vi "pruebas con Alarm Log y Fill Table.vi"() -> ()   [LabVIEW 2018]
panel:
  in  "Filtrar por Alarma?":bool
  out "Array":string[][](array[string])
  out "Real Time Alarms (last 100 records)":i32(listbox)
  out "RT Alarm Log":string[](array[string])
  out "Numeric":i32
  out "PQ_Log array out":i16[](array[numeric])
  out "Boolean array 6":bool[](array[boolean])
  in  "stop":bool
  # "Sag_Indication_Detected"
  # "Swell_Indication_Detected"
  # "Transient_Indication"
  # "200mS_Sag_Swell_Status_Flag"
  # "3s_Sag_Swell_Status_Flag"
  # "10m_Sag_Swell_Status_Flag"
  # "2h_Sag_Swell_Status_Flag"
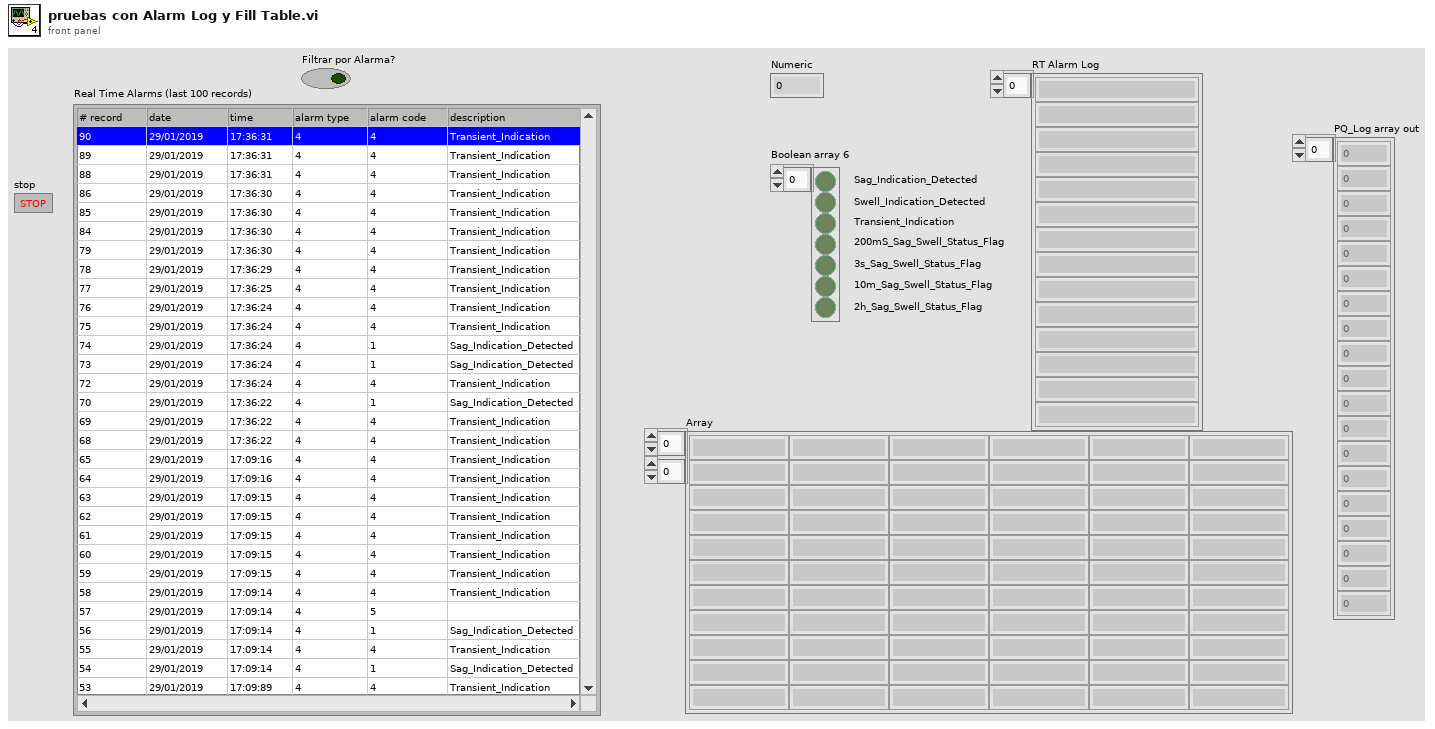
[diagram p1: front panel]
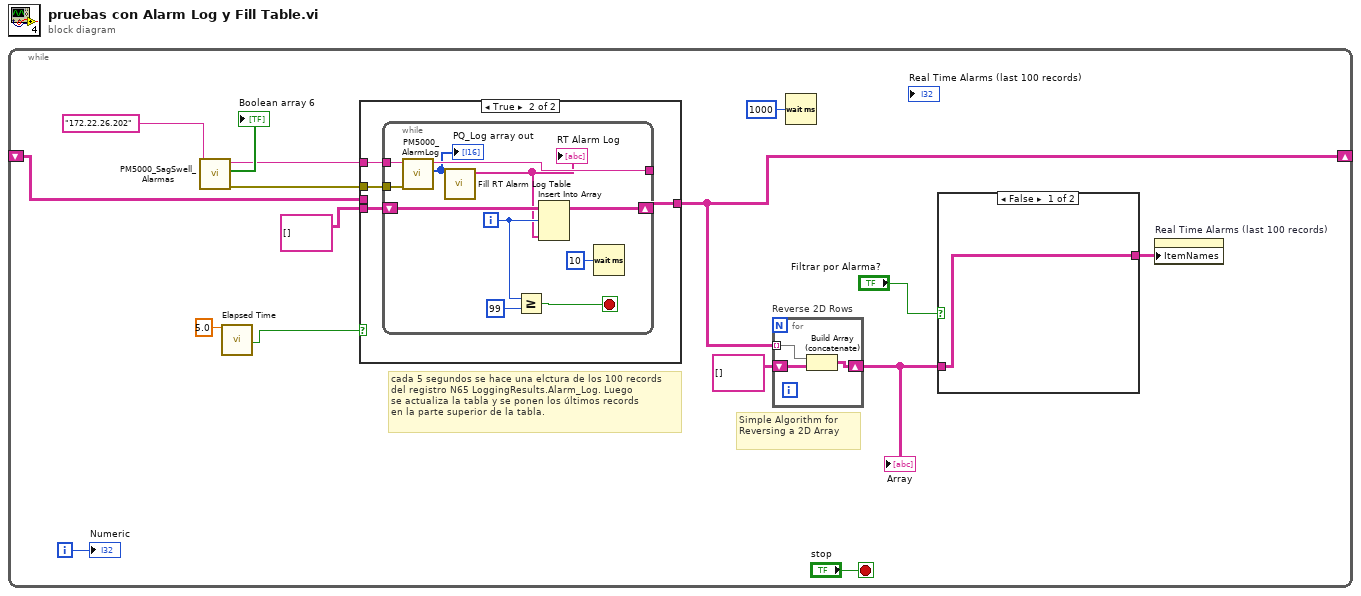
[diagram p0: block diagram]
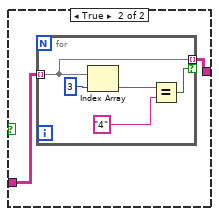
[diagram p2: hidden frame]
diagram:
  n1 = while {
    shift-right: [w4] -> _
    shift-left: _ -> [w6]
    i -> [w10]
    stop <- "stop" stop-if-true
    # "Simple Algorithm for Reversing a 2D Array"
    # "cada 5 segundos se hace una elctura de los 100 records\ndel registro N65 LoggingResults.Alarm_Log. Luego\nse actualiza la tabla y se ponen los últimos records \nen la parte superior de la tabla."
    n2 = call "PM5000_SagSwell_Alarmas.vi"("Network Path"="172.22.26.202") -> ("error out"=w11:errorcluster, "PQ_Alarmas"=→"Boolean array 6":bool[], "Network Path out"=w12:string)  [unwired: 8 in]
    n3 = call "Elapsed Time"("Time Target (s)"=5.0) -> ("Time has Elapsed"=w7:bool)  [unwired: 11 in, 7 out]
    n4 = case shown="True" w7 {
      tunnel: w12 -> [_ w32]
      tunnel: w11 -> [_ w31]
      tunnel: string[][] [] -> [_ w30]
      tunnel: [w28 w29] -> w4
      tunnel: w6 -> [w28 _]
      frame False {
      }
      frame True {
        n5 = while {
          tunnel: w32 -> [w43]
          tunnel: w31 -> [w42]
          tunnel: [w41] -> _
          shift-right: [w39] -> w29
          shift-left: w30 -> [w40]
          i -> [w38]
          stop <- w36 stop-if-true
          n6 = call "PM5000_AlarmLog.vi"("error in"=w42, "Network Path"=w43) -> ("Alarm Log"=w34:i16[], "Network Path out"=w41:string)  [unwired: 7 in, 1 out]
          "PQ_Log array out" <- w34
          n7 = call "Fill RT Alarm Log Table.vi"("Alarm Log"=w34) -> ("appended array"=w33:string[])  [unwired: 10 in]
          "RT Alarm Log" <- w33
          n8 = Greater Or Equal?(x=w38, y=99) -> (x >= y?=w36:bool)
          n9 = Insert Into Array(array=w40, index (row)=w38, new element=w33) -> (w39:string[][])  [unwired: 1 in]
          n10 = Wait (ms)(milliseconds to wait=u32 10) -> ()  [unwired: 1 out]
        }
      }
    }
    n11 = for "Reverse 2D Rows" {
      tunnel: w4 -> [w27] mode=indexing
      shift-right: [w25] -> w3
      shift-left: string[][] [] -> [w26]
      n12 = Build Array (concatenate)(w27, w26) -> (w25:string[][])
    }
    "Array" <- w3
    n13 = Wait (ms)(milliseconds to wait=u32 1000) -> ()  [unwired: 1 out]
    n14 = case shown="False" "Filtrar por Alarma?" {
      tunnel: w3 -> [w17 w19]
      tunnel: [w17 w18] -> w2
      frame False {
      }
      frame True {
        n15 = for {
          tunnel: w19 -> [w24] mode=indexing
          tunnel: [w24] -> w18 mode=indexing if=w20
          n16 = Index Array(array=w24, index=3) -> (element=w22:string)
          n17 = Equal?(x=w22, y="4" ("Filtro")) -> (x = y?=w20:bool)
        }
      }
    }
    n18 = property on="Real Time Alarms (last 100 records)" class="MCListbox (strict)"("ItemNames"=w2) -> ()  [unwired: 2 in, 2 out]
    "Numeric" <- w10
  }
